vi "Autonomous Independent.vi"() -> ()   [LabVIEW 2012]
doc: "This VI is called when autonomous begins, and will automatically be terminated when autonomous ends. You can carry out timed or sensor driven robot movement independently without needing to return to the caller."
uses:
  Robot Global Data.vi
  <vilib>/Rock Robotics/WPI/RobotDrive/WPI_RobotDriveGetSetRefNum.vi
  <vilib>/Rock Robotics/WPI/Joystick/WPI_JoystickGetSetRefNum.vi
  <vilib>/Rock Robotics/WPI/RobotDrive/WPI_RobotDriveArcadeDrive_Standard(NoSaturation).vi
panel:
  out "Current Movement, for debugging":T1 {"Y Joystick Value" scale=1.0..-1.0; "X Joystick Value" scale=-1.0..1.0}
  in  "Array of robot movements":T2(array[cluster]) {"Y Joystick Value" scale=1.0..-1.0; "X Joystick Value" scale=-1.0..1.0}
  # "Be sure to right-click and choose Data Operations>>Make Current Value default if you want to save the array values with the VI"
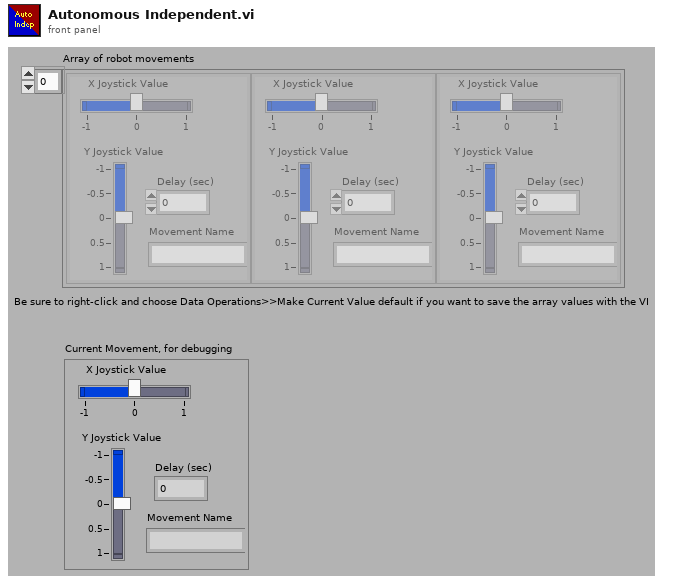
[diagram p1: front panel]
types:
  T1 = cluster{"X Joystick Value":dbl, "Y Joystick Value":dbl, "Delay (sec)":dbl, "Movement Name":string}
  T2 = cluster{"X Joystick Value":dbl, "Y Joystick Value":dbl, "Delay (sec)":dbl, "Movement Name":string}[]
  T3 = typedef "WPI_JoystickDevRef.ctl" = cluster{"Device":T4}
  T4 = typedef "WPI_JoystickDeviceEnum.ctl" = enum16{"USB 1", "USB 2", "USB 3", "USB 4", "Kinect 1", "Kinect 2"}
  T5 = cluster{"axis 1 (x)":dbl, "axis 2 (y)":dbl, "axis 3 (throttle)":dbl, "axis 4":dbl, "axis 5":dbl, "axis 6":dbl}
  T6 = typedef "WPI_RobotDriveDevRef.ctl" = cluster{"DevStatus":errorcluster, "Motors[]":T7[], "Square Inputs":bool, "Max Output":dbl, "Isochronous":bool}
  T7 = typedef "WPI_MotorControlDeviceRef.ctl" = cluster{"DeviceStatus":errorcluster, "Type":enum16{"PWM", "CAN"}, "PWM":cluster{"Digital Module":T8, "PWM Channel":T9, "DeadBand":T10}, "CAN":cluster{"Device Number":u8, "Control Mode":T11, "Semaphore":T12, "Max Vout":dbl}, "Invert":bool, "TransformRef":T13, "InvTransformRef":T13}
  T8 = typedef "FPGA_TypedefDigitalModule.ctl" = enum16{"Digital Module 1", "Digital Module 2"}
  T9 = typedef "FPGA_DIOPWMChannel.ctl" = enum8{"PWM 1", "PWM 2", "PWM 3", "PWM 4", "PWM 5", "PWM 6", "PWM 7", "PWM 8", "PWM 9", "PWM 10", "Invalid"}
  T10 = typedef "WPI_PWMDeadband.ctl" = cluster{"Name":string, "maxPositivePwm":i32, "minPositivePwm":i32, "centerPwm":i32, "maxNegativePwm":i32, "minNegativePwm":i32, "angularRange":u16}
  T11 = typedef "WPI_CANJaguar_ControlMode.ctl" = enum8{"Percent VBus", "Current", "Speed", "Position", "Voltage"}
  T12 = typedef "Semaphore RefNum" = refnum<k1>
  T13 = typedef "WPI_PWMTransform_ConPane.ctl" = refnum<vi>
  T14 = typedef "WPI_ServoDeviceRef.ctl" = cluster{"DeviceStatus":errorcluster, "Digital Module":T8, "PWM Channel":T9, "DeadBand":T10}
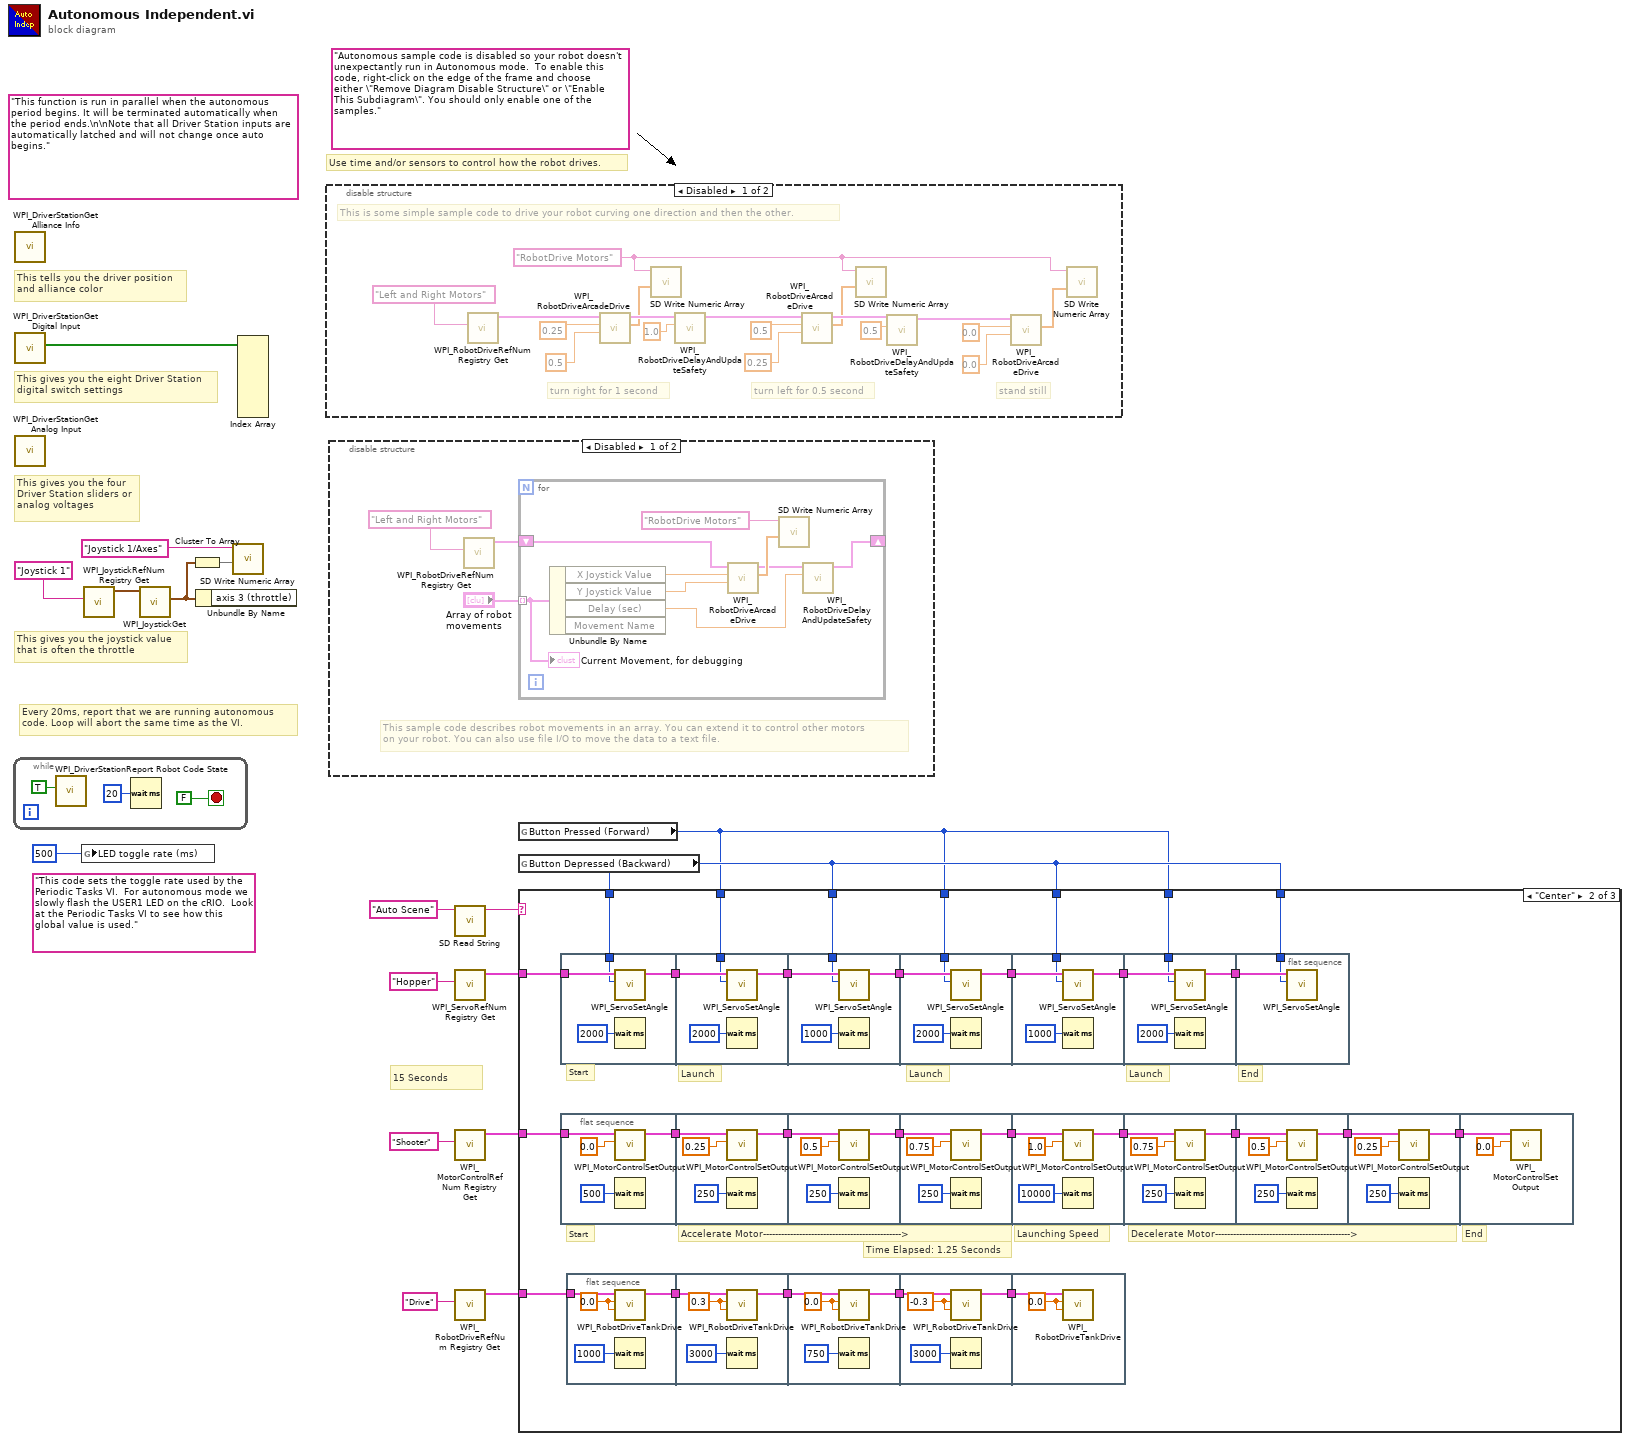
[diagram p0: block diagram]
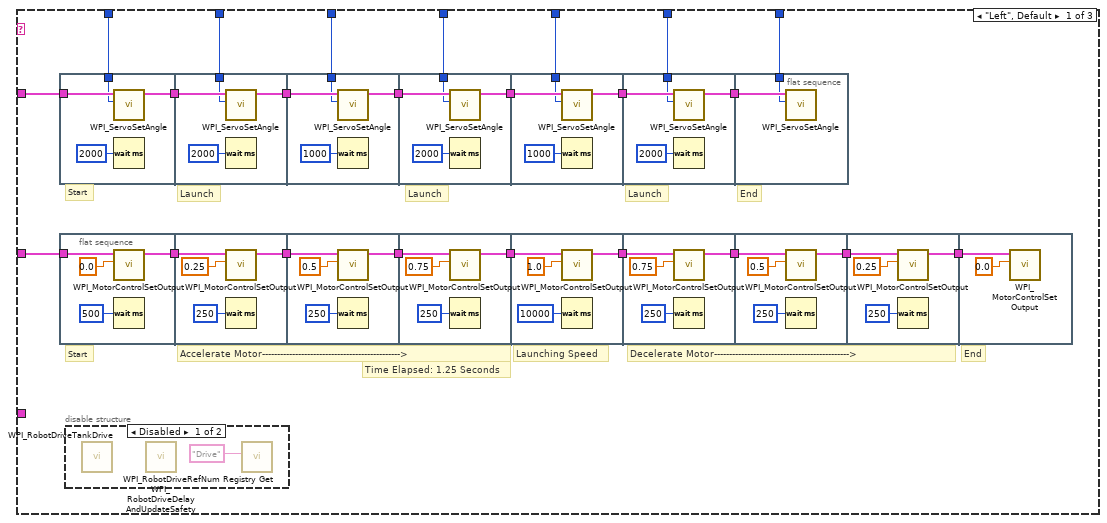
[diagram p2: hidden frame]
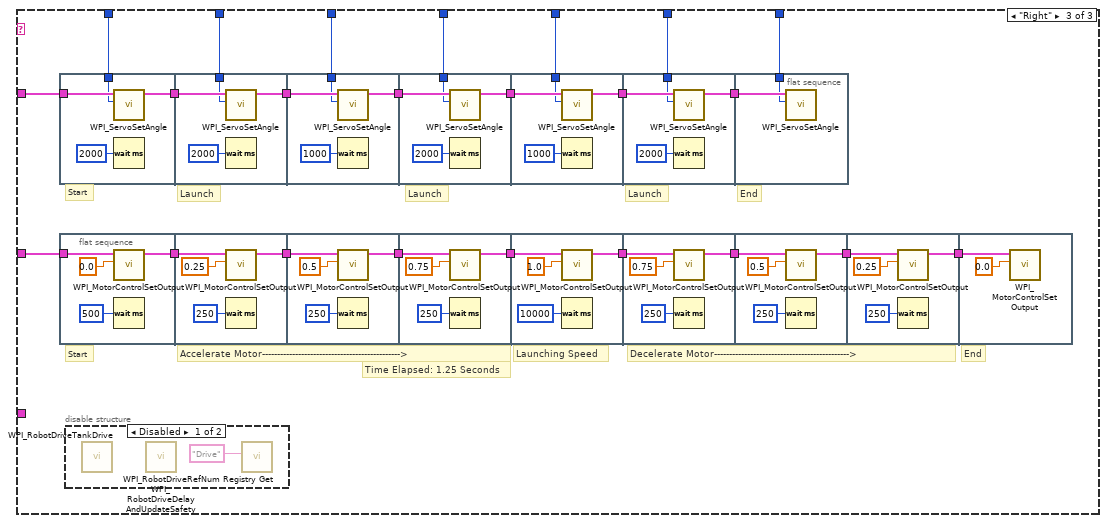
[diagram p4: hidden frame]
diagram:
  (unwired) "This code sets the toggle rate used by the Periodic Tasks VI.  For autonomous mode we slowly flash the USER1 LED on the cRIO.  Look at the Periodic Tasks VI to see how this global value is used."
  (unwired) "Autonomous sample code is disabled so your robot doesn't unexpectantly run in Autonomous mode.  To enable this code, right-click on the edge of the frame and choose either \"Remove Diagram Disable Structure\" or \"Enable This Subdiagram\". You should only enable one of the samples."
  (unwired) "This function is run in parallel when the autonomous period begins. It will be terminated automatically when the period ends.\n\nNote that all Driver Station inputs are automatically latched and will not change once auto begins."
  # "15 Seconds"
  # "Every 20ms, report that we are running autonomous\ncode. Loop will abort the same time as the VI."
  # "This gives you the joystick value\nthat is often the throttle"
  # "Use time and/or sensors to control how the robot drives."
  # "This tells you the driver position\nand alliance color"
  # "This gives you the eight Driver Station\ndigital switch settings"
  # "This gives you the four\nDriver Station sliders or\nanalog voltages"
  n1 = while {
    stop <- FALSE stop-if-true
    n2 = call <vilib>:"WPI_DriverStationReport Robot Code State.vi"("Autonomous"=TRUE) -> ()  [unwired: 10 in, 1 out]
    n3 = Wait (ms)(milliseconds to wait=u32 20) -> ()  [unwired: 1 out]
  }
  n4 = call <vilib>:"WPI_DriverStationGet Alliance Info.vi"() -> ()  [unwired: 12 out]
  n5 = call <vilib>:"WPI_DriverStationGet Digital Input.vi"() -> ("Driver Station Digital Input (1-8)"=w17:bool[])  [unwired: 11 out]
  n6 = call <vilib>:"WPI_DriverStationGet Analog Input.vi"() -> ()  [unwired: 12 out]
  n7 = global write "Robot Global Data.vi" "LED toggle rate (ms)"(u32 500 ("LED ms toggle rate")) -> ()
  n8 = call <vilib>:"WPI_JoystickRefNum Registry Get.vi"("refnum name"="Joystick 1") -> ("JoystickDevRef"=w15:T3)  [unwired: 1 in, 9 out]
  n9 = call <vilib>:"WPI_JoystickGet.vi"("JoystickDevRef"=w15) -> ("Axes"=w12:T5)  [unwired: 1 in, 5 out]
  n10 = Cluster To Array(cluster=w12) -> (array=w13:dbl[])
  n11 = Unbundle By Name(w12) -> ()  [unwired: 1 out]
  n12 = call <vilib>:"SD Write Numeric Array.vi"("Numeric Array"=w13, "Name"="Joystick 1/Axes") -> ()  [unwired: 8 in, 2 out]
  n13 = Index Array(array=w17) -> ()  [unwired: 8 in, 8 out]
  n14 = disable-structure shown="Disabled" {
    frame Disabled {
      w21 = "RobotDrive Motors" ("Name")
      # "This is some simple sample code to drive your robot curving one direction and then the other."
      # "stand still"
      # "turn left for 0.5 second"
      # "turn right for 1 second"
      n15 = call <vilib>:"WPI_RobotDriveRefNum Registry Get.vi"("refnum name"="Left and Right Motors") -> ("RobotDriveDevRef"=w25:T6)  [unwired: 1 in, 9 out]
      n16 = call-poly <vilib>:"WPI_RobotDriveArcadeDrive.vi"("Y axis value"=0.5 ("X axis value"), "X axis value"=0.25, "RobotDriveDevRef"=w25) -> ("Motor Values"=w24:dbl[], "RobotDriveDevRef"=w32:T6)  [unwired: 1 in, 6 out]
      n17 = call <vilib>:"SD Write Numeric Array.vi"("Numeric Array"=w24, "Name"=w21) -> ()  [unwired: 8 in, 2 out]
      n18 = call <vilib>:"WPI_RobotDriveDelayAndUpdateSafety.vi"("Delay (s)"=1.0, "RobotDriveDevRef"=w32) -> ("RobotDriveDevRef 2"=w31:T6)  [unwired: 8 in, 1 out]
      n19 = call-poly <vilib>:"WPI_RobotDriveArcadeDrive.vi"("Y axis value"=0.25 ("X axis value"), "X axis value"=0.5, "RobotDriveDevRef"=w31) -> ("Motor Values"=w23:dbl[], "RobotDriveDevRef"=w30:T6)  [unwired: 1 in, 6 out]
      n20 = call <vilib>:"SD Write Numeric Array.vi"("Numeric Array"=w23, "Name"=w21) -> ()  [unwired: 8 in, 2 out]
      n21 = call <vilib>:"WPI_RobotDriveDelayAndUpdateSafety.vi"("Delay (s)"=0.5, "RobotDriveDevRef"=w30) -> ("RobotDriveDevRef 2"=w29:T6)  [unwired: 8 in, 1 out]
      n22 = call-poly <vilib>:"WPI_RobotDriveArcadeDrive.vi"("Y axis value"=0.0 ("X axis value"), "X axis value"=0.0, "RobotDriveDevRef"=w29) -> ("Motor Values"=w22:dbl[])  [unwired: 1 in, 7 out]
      n23 = call <vilib>:"SD Write Numeric Array.vi"("Numeric Array"=w22, "Name"=w21) -> ()  [unwired: 8 in, 2 out]
    }
    frame Enabled {
    }
  }
  n24 = disable-structure shown="Disabled" {
    frame Disabled {
      # "This sample code describes robot movements in an array. You can extend it to control other motors\non your robot. You can also use file I/O to move the data to a text file."
      n25 = call <vilib>:"WPI_RobotDriveRefNum Registry Get.vi"("refnum name"="Left and Right Motors") -> ("RobotDriveDevRef"=w40:T6)  [unwired: 1 in, 9 out]
      n26 = for {
        shift-right: [w46] -> _
        shift-left: w40 -> [w47]
        tunnel: "Array of robot movements" -> [w42] mode=indexing
        n27 = Unbundle By Name(w42) -> ("X Joystick Value"=w45:dbl, "Y Joystick Value"=w44:dbl, "Delay (sec)"=w43:dbl)  [unwired: 1 out]
        n28 = call-poly <vilib>:"WPI_RobotDriveArcadeDrive.vi"("Y axis value"=w44, "X axis value"=w45, "RobotDriveDevRef"=w47) -> ("Motor Values"=w49:dbl[], "RobotDriveDevRef"=w48:T6)  [unwired: 1 in, 6 out]
        n29 = call <vilib>:"SD Write Numeric Array.vi"("Numeric Array"=w49, "Name"="RobotDrive Motors") -> ()  [unwired: 8 in, 2 out]
        n30 = call <vilib>:"WPI_RobotDriveDelayAndUpdateSafety.vi"("Delay (s)"=w43, "RobotDriveDevRef"=w48) -> ("RobotDriveDevRef 2"=w46:T6)  [unwired: 8 in, 1 out]
        "Current Movement, for debugging" <- w42
      }
    }
    frame Enabled {
    }
  }
  n31 = call <vilib>:"SD Read String.vi"("Name"="Auto Scene") -> ("String"=w6:string)  [unwired: 8 in, 2 out]
  n32 = call <vilib>:"WPI_ServoRefNum Registry Get.vi"("refnum name"="Hopper") -> ("ServoDeviceRef"=w8:T14)  [unwired: 9 in, 1 out]
  n33 = call <vilib>:"WPI_MotorControlRefNum Registry Get.vi"("refnum name"="Shooter") -> ("MotorControlDevRef"=w9:T7)  [unwired: 9 in, 1 out]
  n34 = call <vilib>:"WPI_RobotDriveRefNum Registry Get.vi"("refnum name"="Drive") -> ("RobotDriveDevRef"=w1:T6)  [unwired: 9 in, 1 out]
  n35 = global read "Robot Global Data.vi" "Button Pressed (Forward)"() -> (w3:i32)
  n36 = global read "Robot Global Data.vi" "Button Depressed (Backward)"() -> (w4:i32)
  n37 = case shown="\"Center\"" w6 {
    tunnel: w9 -> [w73 w148 w249]
    tunnel: w8 -> [w71 w147 w248]
    tunnel: w4 -> [w57 w146 w241]
    tunnel: w4 -> [w56 w144 w243]
    tunnel: w4 -> [w55 w142 w245]
    tunnel: w4 -> [w54 w140 w247]
    tunnel: w3 -> [w53 w145 w242]
    tunnel: w3 -> [w52 w143 w244]
    tunnel: w3 -> [w51 w141 w246]
    tunnel: w1 -> [_ w139 _]
    frame "Left", Default {
      # "Time Elapsed: 1.25 Seconds"
      # "End"
      # "Decelerate Motor--------------------------------------------->"
      # "Accelerate Motor---------------------------------------------->"
      # "Launching Speed"
      # "Start"
      # "End"
      # "Launch"
      # "Launch"
      # "Launch"
      # "Start"
      n38 = flat-sequence {
        tunnel: w71 -> [w78]
        tunnel: [w77] -> w70
        tunnel: w57 -> [w75]
        tunnel: w70 -> [w82]
        tunnel: [w80] -> w65
        tunnel: w53 -> [w79]
        tunnel: [w85] -> w69
        tunnel: w65 -> [w86]
        tunnel: w56 -> [w83]
        tunnel: w69 -> [w90]
        tunnel: [w89] -> w68
        tunnel: w52 -> [w87]
        tunnel: w68 -> [w94]
        tunnel: [w93] -> w67
        tunnel: w55 -> [w91]
        tunnel: w67 -> [w98]
        tunnel: [w97] -> w66
        tunnel: w51 -> [w95]
        tunnel: w66 -> [w100]
        tunnel: w54 -> [w99]
        frame #0 {
          n39 = call <vilib>:"WPI_ServoSetAngle.vi"("Angle"=w75, "ServoDeviceRef"=w78) -> ("ServoDeviceRef"=w77:T14)  [unwired: 8 in, 1 out]
          n40 = Wait (ms)(milliseconds to wait=u32 2000) -> ()  [unwired: 1 out]
        }
        frame #1 {
          n41 = call <vilib>:"WPI_ServoSetAngle.vi"("Angle"=w79, "ServoDeviceRef"=w82) -> ("ServoDeviceRef"=w80:T14)  [unwired: 8 in, 1 out]
          n42 = Wait (ms)(milliseconds to wait=u32 2000) -> ()  [unwired: 1 out]
        }
        frame #2 {
          n43 = call <vilib>:"WPI_ServoSetAngle.vi"("Angle"=w83, "ServoDeviceRef"=w86) -> ("ServoDeviceRef"=w85:T14)  [unwired: 8 in, 1 out]
          n44 = Wait (ms)(milliseconds to wait=u32 1000) -> ()  [unwired: 1 out]
        }
        frame #3 {
          n45 = call <vilib>:"WPI_ServoSetAngle.vi"("Angle"=w87, "ServoDeviceRef"=w90) -> ("ServoDeviceRef"=w89:T14)  [unwired: 8 in, 1 out]
          n46 = Wait (ms)(milliseconds to wait=u32 2000) -> ()  [unwired: 1 out]
        }
        frame #4 {
          n47 = call <vilib>:"WPI_ServoSetAngle.vi"("Angle"=w91, "ServoDeviceRef"=w94) -> ("ServoDeviceRef"=w93:T14)  [unwired: 8 in, 1 out]
          n48 = Wait (ms)(milliseconds to wait=u32 1000) -> ()  [unwired: 1 out]
        }
        frame #5 {
          n49 = call <vilib>:"WPI_ServoSetAngle.vi"("Angle"=w95, "ServoDeviceRef"=w98) -> ("ServoDeviceRef"=w97:T14)  [unwired: 8 in, 1 out]
          n50 = Wait (ms)(milliseconds to wait=u32 2000) -> ()  [unwired: 1 out]
        }
        frame #6 {
          n51 = call <vilib>:"WPI_ServoSetAngle.vi"("Angle"=w99, "ServoDeviceRef"=w100) -> ()  [unwired: 8 in, 2 out]
        }
      }
      n52 = flat-sequence {
        tunnel: w73 -> [w104]
        tunnel: [w102] -> w72
        tunnel: w72 -> [w107]
        tunnel: [w105] -> w64
        tunnel: w64 -> [w110]
        tunnel: [w109] -> w63
        tunnel: w63 -> [w114]
        tunnel: [w113] -> w62
        tunnel: w62 -> [w118]
        tunnel: [w117] -> w61
        tunnel: w61 -> [w122]
        tunnel: [w121] -> w60
        tunnel: w60 -> [w126]
        tunnel: [w125] -> w59
        tunnel: w59 -> [w130]
        tunnel: [w129] -> w58
        tunnel: w58 -> [w133]
        frame #0 {
          n53 = call <vilib>:"WPI_MotorControlSetOutput.vi"("Output"=0.0, "MotorControlDevRef"=w104) -> ("MotorControlDevRef"=w102:T7)  [unwired: 7 in, 2 out]
          n54 = Wait (ms)(milliseconds to wait=u32 500) -> ()  [unwired: 1 out]
        }
        frame #1 {
          n55 = call <vilib>:"WPI_MotorControlSetOutput.vi"("Output"=0.25, "MotorControlDevRef"=w107) -> ("MotorControlDevRef"=w105:T7)  [unwired: 7 in, 2 out]
          n56 = Wait (ms)(milliseconds to wait=u32 250) -> ()  [unwired: 1 out]
        }
        frame #2 {
          n57 = call <vilib>:"WPI_MotorControlSetOutput.vi"("Output"=0.5, "MotorControlDevRef"=w110) -> ("MotorControlDevRef"=w109:T7)  [unwired: 7 in, 2 out]
          n58 = Wait (ms)(milliseconds to wait=u32 250) -> ()  [unwired: 1 out]
        }
        frame #3 {
          n59 = call <vilib>:"WPI_MotorControlSetOutput.vi"("Output"=0.75, "MotorControlDevRef"=w114) -> ("MotorControlDevRef"=w113:T7)  [unwired: 7 in, 2 out]
          n60 = Wait (ms)(milliseconds to wait=u32 250) -> ()  [unwired: 1 out]
        }
        frame #4 {
          n61 = call <vilib>:"WPI_MotorControlSetOutput.vi"("Output"=1.0, "MotorControlDevRef"=w118) -> ("MotorControlDevRef"=w117:T7)  [unwired: 7 in, 2 out]
          n62 = Wait (ms)(milliseconds to wait=u32 10000) -> ()  [unwired: 1 out]
        }
        frame #5 {
          n63 = call <vilib>:"WPI_MotorControlSetOutput.vi"("Output"=0.75, "MotorControlDevRef"=w122) -> ("MotorControlDevRef"=w121:T7)  [unwired: 7 in, 2 out]
          n64 = Wait (ms)(milliseconds to wait=u32 250) -> ()  [unwired: 1 out]
        }
        frame #6 {
          n65 = call <vilib>:"WPI_MotorControlSetOutput.vi"("Output"=0.5, "MotorControlDevRef"=w126) -> ("MotorControlDevRef"=w125:T7)  [unwired: 7 in, 2 out]
          n66 = Wait (ms)(milliseconds to wait=u32 250) -> ()  [unwired: 1 out]
        }
        frame #7 {
          n67 = call <vilib>:"WPI_MotorControlSetOutput.vi"("Output"=0.25, "MotorControlDevRef"=w130) -> ("MotorControlDevRef"=w129:T7)  [unwired: 7 in, 2 out]
          n68 = Wait (ms)(milliseconds to wait=u32 250) -> ()  [unwired: 1 out]
        }
        frame #8 {
          n69 = call <vilib>:"WPI_MotorControlSetOutput.vi"("Output"=0.0, "MotorControlDevRef"=w133) -> ()  [unwired: 7 in, 3 out]
        }
      }
      n70 = disable-structure shown="Disabled" {
        frame Disabled {
          n71 = call <vilib>:"WPI_RobotDriveTankDrive.vi"() -> ()  [unwired: 9 in, 3 out]
          n72 = call <vilib>:"WPI_RobotDriveDelayAndUpdateSafety.vi"() -> ()  [unwired: 10 in, 2 out]
          n73 = call <vilib>:"WPI_RobotDriveRefNum Registry Get.vi"("refnum name"="Drive") -> ()  [unwired: 9 in, 2 out]
        }
        frame Enabled {
        }
      }
    }
    frame "Center" {
      # "Time Elapsed: 1.25 Seconds"
      # "End"
      # "Decelerate Motor--------------------------------------------->"
      # "Accelerate Motor---------------------------------------------->"
      # "Launching Speed"
      # "Start"
      # "End"
      # "Launch"
      # "Launch"
      # "Launch"
      # "Start"
      n74 = flat-sequence {
        tunnel: w147 -> [w184]
        tunnel: [w183] -> w154
        tunnel: w146 -> [w181]
        tunnel: w154 -> [w188]
        tunnel: [w186] -> w153
        tunnel: w145 -> [w185]
        tunnel: [w191] -> w152
        tunnel: w153 -> [w192]
        tunnel: w144 -> [w189]
        tunnel: w152 -> [w196]
        tunnel: [w195] -> w151
        tunnel: w143 -> [w193]
        tunnel: w151 -> [w200]
        tunnel: [w199] -> w150
        tunnel: w142 -> [w197]
        tunnel: w150 -> [w204]
        tunnel: [w203] -> w149
        tunnel: w141 -> [w201]
        tunnel: w149 -> [w206]
        tunnel: w140 -> [w205]
        frame #0 {
          n75 = call <vilib>:"WPI_ServoSetAngle.vi"("Angle"=w181, "ServoDeviceRef"=w184) -> ("ServoDeviceRef"=w183:T14)  [unwired: 8 in, 1 out]
          n76 = Wait (ms)(milliseconds to wait=u32 2000) -> ()  [unwired: 1 out]
        }
        frame #1 {
          n77 = call <vilib>:"WPI_ServoSetAngle.vi"("Angle"=w185, "ServoDeviceRef"=w188) -> ("ServoDeviceRef"=w186:T14)  [unwired: 8 in, 1 out]
          n78 = Wait (ms)(milliseconds to wait=u32 2000) -> ()  [unwired: 1 out]
        }
        frame #2 {
          n79 = call <vilib>:"WPI_ServoSetAngle.vi"("Angle"=w189, "ServoDeviceRef"=w192) -> ("ServoDeviceRef"=w191:T14)  [unwired: 8 in, 1 out]
          n80 = Wait (ms)(milliseconds to wait=u32 1000) -> ()  [unwired: 1 out]
        }
        frame #3 {
          n81 = call <vilib>:"WPI_ServoSetAngle.vi"("Angle"=w193, "ServoDeviceRef"=w196) -> ("ServoDeviceRef"=w195:T14)  [unwired: 8 in, 1 out]
          n82 = Wait (ms)(milliseconds to wait=u32 2000) -> ()  [unwired: 1 out]
        }
        frame #4 {
          n83 = call <vilib>:"WPI_ServoSetAngle.vi"("Angle"=w197, "ServoDeviceRef"=w200) -> ("ServoDeviceRef"=w199:T14)  [unwired: 8 in, 1 out]
          n84 = Wait (ms)(milliseconds to wait=u32 1000) -> ()  [unwired: 1 out]
        }
        frame #5 {
          n85 = call <vilib>:"WPI_ServoSetAngle.vi"("Angle"=w201, "ServoDeviceRef"=w204) -> ("ServoDeviceRef"=w203:T14)  [unwired: 8 in, 1 out]
          n86 = Wait (ms)(milliseconds to wait=u32 2000) -> ()  [unwired: 1 out]
        }
        frame #6 {
          n87 = call <vilib>:"WPI_ServoSetAngle.vi"("Angle"=w205, "ServoDeviceRef"=w206) -> ()  [unwired: 8 in, 2 out]
        }
      }
      n88 = flat-sequence {
        tunnel: w148 -> [w210]
        tunnel: [w208] -> w162
        tunnel: w162 -> [w213]
        tunnel: [w211] -> w161
        tunnel: w161 -> [w216]
        tunnel: [w215] -> w160
        tunnel: w160 -> [w220]
        tunnel: [w219] -> w159
        tunnel: w159 -> [w224]
        tunnel: [w223] -> w158
        tunnel: w158 -> [w228]
        tunnel: [w227] -> w157
        tunnel: w157 -> [w232]
        tunnel: [w231] -> w156
        tunnel: w156 -> [w236]
        tunnel: [w235] -> w155
        tunnel: w155 -> [w239]
        frame #0 {
          n89 = call <vilib>:"WPI_MotorControlSetOutput.vi"("Output"=0.0, "MotorControlDevRef"=w210) -> ("MotorControlDevRef"=w208:T7)  [unwired: 7 in, 2 out]
          n90 = Wait (ms)(milliseconds to wait=u32 500) -> ()  [unwired: 1 out]
        }
        frame #1 {
          n91 = call <vilib>:"WPI_MotorControlSetOutput.vi"("Output"=0.25, "MotorControlDevRef"=w213) -> ("MotorControlDevRef"=w211:T7)  [unwired: 7 in, 2 out]
          n92 = Wait (ms)(milliseconds to wait=u32 250) -> ()  [unwired: 1 out]
        }
        frame #2 {
          n93 = call <vilib>:"WPI_MotorControlSetOutput.vi"("Output"=0.5, "MotorControlDevRef"=w216) -> ("MotorControlDevRef"=w215:T7)  [unwired: 7 in, 2 out]
          n94 = Wait (ms)(milliseconds to wait=u32 250) -> ()  [unwired: 1 out]
        }
        frame #3 {
          n95 = call <vilib>:"WPI_MotorControlSetOutput.vi"("Output"=0.75, "MotorControlDevRef"=w220) -> ("MotorControlDevRef"=w219:T7)  [unwired: 7 in, 2 out]
          n96 = Wait (ms)(milliseconds to wait=u32 250) -> ()  [unwired: 1 out]
        }
        frame #4 {
          n97 = call <vilib>:"WPI_MotorControlSetOutput.vi"("Output"=1.0, "MotorControlDevRef"=w224) -> ("MotorControlDevRef"=w223:T7)  [unwired: 7 in, 2 out]
          n98 = Wait (ms)(milliseconds to wait=u32 10000) -> ()  [unwired: 1 out]
        }
        frame #5 {
          n99 = call <vilib>:"WPI_MotorControlSetOutput.vi"("Output"=0.75, "MotorControlDevRef"=w228) -> ("MotorControlDevRef"=w227:T7)  [unwired: 7 in, 2 out]
          n100 = Wait (ms)(milliseconds to wait=u32 250) -> ()  [unwired: 1 out]
        }
        frame #6 {
          n101 = call <vilib>:"WPI_MotorControlSetOutput.vi"("Output"=0.5, "MotorControlDevRef"=w232) -> ("MotorControlDevRef"=w231:T7)  [unwired: 7 in, 2 out]
          n102 = Wait (ms)(milliseconds to wait=u32 250) -> ()  [unwired: 1 out]
        }
        frame #7 {
          n103 = call <vilib>:"WPI_MotorControlSetOutput.vi"("Output"=0.25, "MotorControlDevRef"=w236) -> ("MotorControlDevRef"=w235:T7)  [unwired: 7 in, 2 out]
          n104 = Wait (ms)(milliseconds to wait=u32 250) -> ()  [unwired: 1 out]
        }
        frame #8 {
          n105 = call <vilib>:"WPI_MotorControlSetOutput.vi"("Output"=0.0, "MotorControlDevRef"=w239) -> ()  [unwired: 7 in, 3 out]
        }
      }
      n106 = flat-sequence {
        tunnel: w139 -> [w164]
        tunnel: [w163] -> w138
        tunnel: w138 -> [w168]
        tunnel: [w167] -> w137
        tunnel: w137 -> [w172]
        tunnel: [w171] -> w136
        tunnel: w136 -> [w176]
        tunnel: [w175] -> w135
        tunnel: w135 -> [w179]
        frame #0 {
          w165 = 0.0 ("Left axis value")
          n107 = call <vilib>:"WPI_RobotDriveTankDrive.vi"("Right axis value"=w165, "Left axis value"=w165, "RobotDriveDevRef"=w164) -> ("RobotDriveDevRef"=w163:T6)  [unwired: 6 in, 2 out]
          n108 = Wait (ms)(milliseconds to wait=u32 1000) -> ()  [unwired: 1 out]
        }
        frame #1 {
          w169 = 0.3 ("Left axis value")
          n109 = call <vilib>:"WPI_RobotDriveTankDrive.vi"("Right axis value"=w169, "Left axis value"=w169, "RobotDriveDevRef"=w168) -> ("RobotDriveDevRef"=w167:T6)  [unwired: 6 in, 2 out]
          n110 = Wait (ms)(milliseconds to wait=u32 3000) -> ()  [unwired: 1 out]
        }
        frame #2 {
          w173 = 0.0 ("Left axis value")
          n111 = call <vilib>:"WPI_RobotDriveTankDrive.vi"("Right axis value"=w173, "Left axis value"=w173, "RobotDriveDevRef"=w172) -> ("RobotDriveDevRef"=w171:T6)  [unwired: 6 in, 2 out]
          n112 = Wait (ms)(milliseconds to wait=u32 750) -> ()  [unwired: 1 out]
        }
        frame #3 {
          w178 = -0.3 ("Left axis value")
          n113 = call <vilib>:"WPI_RobotDriveTankDrive.vi"("Right axis value"=w178, "Left axis value"=w178, "RobotDriveDevRef"=w176) -> ("RobotDriveDevRef"=w175:T6)  [unwired: 6 in, 2 out]
          n114 = Wait (ms)(milliseconds to wait=u32 3000) -> ()  [unwired: 1 out]
        }
        frame #4 {
          w180 = 0.0 ("Left axis value")
          n115 = call <vilib>:"WPI_RobotDriveTankDrive.vi"("Right axis value"=w180, "Left axis value"=w180, "RobotDriveDevRef"=w179) -> ()  [unwired: 6 in, 3 out]
        }
      }
    }
    frame "Right" {
      # "Time Elapsed: 1.25 Seconds"
      # "End"
      # "Decelerate Motor--------------------------------------------->"
      # "Accelerate Motor---------------------------------------------->"
      # "Launching Speed"
      # "Start"
      # "End"
      # "Launch"
      # "Launch"
      # "Launch"
      # "Start"
      n116 = flat-sequence {
        tunnel: w248 -> [w268]
        tunnel: [w267] -> w255
        tunnel: w241 -> [w265]
        tunnel: w255 -> [w272]
        tunnel: [w270] -> w254
        tunnel: w242 -> [w269]
        tunnel: [w275] -> w253
        tunnel: w254 -> [w276]
        tunnel: w243 -> [w273]
        tunnel: w253 -> [w280]
        tunnel: [w279] -> w252
        tunnel: w244 -> [w277]
        tunnel: w252 -> [w284]
        tunnel: [w283] -> w251
        tunnel: w245 -> [w281]
        tunnel: w251 -> [w288]
        tunnel: [w287] -> w250
        tunnel: w246 -> [w285]
        tunnel: w250 -> [w290]
        tunnel: w247 -> [w289]
        frame #0 {
          n117 = call <vilib>:"WPI_ServoSetAngle.vi"("Angle"=w265, "ServoDeviceRef"=w268) -> ("ServoDeviceRef"=w267:T14)  [unwired: 8 in, 1 out]
          n118 = Wait (ms)(milliseconds to wait=u32 2000) -> ()  [unwired: 1 out]
        }
        frame #1 {
          n119 = call <vilib>:"WPI_ServoSetAngle.vi"("Angle"=w269, "ServoDeviceRef"=w272) -> ("ServoDeviceRef"=w270:T14)  [unwired: 8 in, 1 out]
          n120 = Wait (ms)(milliseconds to wait=u32 2000) -> ()  [unwired: 1 out]
        }
        frame #2 {
          n121 = call <vilib>:"WPI_ServoSetAngle.vi"("Angle"=w273, "ServoDeviceRef"=w276) -> ("ServoDeviceRef"=w275:T14)  [unwired: 8 in, 1 out]
          n122 = Wait (ms)(milliseconds to wait=u32 1000) -> ()  [unwired: 1 out]
        }
        frame #3 {
          n123 = call <vilib>:"WPI_ServoSetAngle.vi"("Angle"=w277, "ServoDeviceRef"=w280) -> ("ServoDeviceRef"=w279:T14)  [unwired: 8 in, 1 out]
          n124 = Wait (ms)(milliseconds to wait=u32 2000) -> ()  [unwired: 1 out]
        }
        frame #4 {
          n125 = call <vilib>:"WPI_ServoSetAngle.vi"("Angle"=w281, "ServoDeviceRef"=w284) -> ("ServoDeviceRef"=w283:T14)  [unwired: 8 in, 1 out]
          n126 = Wait (ms)(milliseconds to wait=u32 1000) -> ()  [unwired: 1 out]
        }
        frame #5 {
          n127 = call <vilib>:"WPI_ServoSetAngle.vi"("Angle"=w285, "ServoDeviceRef"=w288) -> ("ServoDeviceRef"=w287:T14)  [unwired: 8 in, 1 out]
          n128 = Wait (ms)(milliseconds to wait=u32 2000) -> ()  [unwired: 1 out]
        }
        frame #6 {
          n129 = call <vilib>:"WPI_ServoSetAngle.vi"("Angle"=w289, "ServoDeviceRef"=w290) -> ()  [unwired: 8 in, 2 out]
        }
      }
      n130 = flat-sequence {
        tunnel: w249 -> [w294]
        tunnel: [w292] -> w263
        tunnel: w263 -> [w297]
        tunnel: [w295] -> w262
        tunnel: w262 -> [w300]
        tunnel: [w299] -> w261
        tunnel: w261 -> [w304]
        tunnel: [w303] -> w260
        tunnel: w260 -> [w308]
        tunnel: [w307] -> w259
        tunnel: w259 -> [w312]
        tunnel: [w311] -> w258
        tunnel: w258 -> [w316]
        tunnel: [w315] -> w257
        tunnel: w257 -> [w320]
        tunnel: [w319] -> w256
        tunnel: w256 -> [w323]
        frame #0 {
          n131 = call <vilib>:"WPI_MotorControlSetOutput.vi"("Output"=0.0, "MotorControlDevRef"=w294) -> ("MotorControlDevRef"=w292:T7)  [unwired: 7 in, 2 out]
          n132 = Wait (ms)(milliseconds to wait=u32 500) -> ()  [unwired: 1 out]
        }
        frame #1 {
          n133 = call <vilib>:"WPI_MotorControlSetOutput.vi"("Output"=0.25, "MotorControlDevRef"=w297) -> ("MotorControlDevRef"=w295:T7)  [unwired: 7 in, 2 out]
          n134 = Wait (ms)(milliseconds to wait=u32 250) -> ()  [unwired: 1 out]
        }
        frame #2 {
          n135 = call <vilib>:"WPI_MotorControlSetOutput.vi"("Output"=0.5, "MotorControlDevRef"=w300) -> ("MotorControlDevRef"=w299:T7)  [unwired: 7 in, 2 out]
          n136 = Wait (ms)(milliseconds to wait=u32 250) -> ()  [unwired: 1 out]
        }
        frame #3 {
          n137 = call <vilib>:"WPI_MotorControlSetOutput.vi"("Output"=0.75, "MotorControlDevRef"=w304) -> ("MotorControlDevRef"=w303:T7)  [unwired: 7 in, 2 out]
          n138 = Wait (ms)(milliseconds to wait=u32 250) -> ()  [unwired: 1 out]
        }
        frame #4 {
          n139 = call <vilib>:"WPI_MotorControlSetOutput.vi"("Output"=1.0, "MotorControlDevRef"=w308) -> ("MotorControlDevRef"=w307:T7)  [unwired: 7 in, 2 out]
          n140 = Wait (ms)(milliseconds to wait=u32 10000) -> ()  [unwired: 1 out]
        }
        frame #5 {
          n141 = call <vilib>:"WPI_MotorControlSetOutput.vi"("Output"=0.75, "MotorControlDevRef"=w312) -> ("MotorControlDevRef"=w311:T7)  [unwired: 7 in, 2 out]
          n142 = Wait (ms)(milliseconds to wait=u32 250) -> ()  [unwired: 1 out]
        }
        frame #6 {
          n143 = call <vilib>:"WPI_MotorControlSetOutput.vi"("Output"=0.5, "MotorControlDevRef"=w316) -> ("MotorControlDevRef"=w315:T7)  [unwired: 7 in, 2 out]
          n144 = Wait (ms)(milliseconds to wait=u32 250) -> ()  [unwired: 1 out]
        }
        frame #7 {
          n145 = call <vilib>:"WPI_MotorControlSetOutput.vi"("Output"=0.25, "MotorControlDevRef"=w320) -> ("MotorControlDevRef"=w319:T7)  [unwired: 7 in, 2 out]
          n146 = Wait (ms)(milliseconds to wait=u32 250) -> ()  [unwired: 1 out]
        }
        frame #8 {
          n147 = call <vilib>:"WPI_MotorControlSetOutput.vi"("Output"=0.0, "MotorControlDevRef"=w323) -> ()  [unwired: 7 in, 3 out]
        }
      }
      n148 = disable-structure shown="Disabled" {
        frame Disabled {
          n149 = call <vilib>:"WPI_RobotDriveTankDrive.vi"() -> ()  [unwired: 9 in, 3 out]
          n150 = call <vilib>:"WPI_RobotDriveDelayAndUpdateSafety.vi"() -> ()  [unwired: 10 in, 2 out]
          n151 = call <vilib>:"WPI_RobotDriveRefNum Registry Get.vi"("refnum name"="Drive") -> ()  [unwired: 9 in, 2 out]
        }
        frame Enabled {
        }
      }
    }
  }
